vi "GetPicture.vi"(8 "ErrorIn":errorcluster, 11 "OpenCVCamIn":refnum<class "OpenCVCam.lvclass">) -> (0 "ErrorOut":errorcluster, 2 "2D Picture":picture, 3 "OpenCVCamOut":refnum<class "OpenCVCam.lvclass">)   [LabVIEW 2021, in "OpenCVCam.lvclass"]
uses:
  OpenCVCam.lvclass
  C:/Localdata/Projects/TriekselSoft/TriekselsoftApplicationFramework/Source/.Externals/Library_TAF/YActor/YActor.lvclass
  .Externals/Library_TAF/YActor/YActor.lvclass/YActor.ctl
  .Externals/Library_TAF/YActor/ExeCmd_sync.vi
  788cf652-cfa8-44ab-bf5d-4ff5bf462e4f.vi
  .Externals/Library_TAF/YActor/private/SendCommand.vi
  .Externals/Library_TAF/YActor/private/WaitForReply.vi
  .Externals/Library_TAF/YActor/private/CreateLocalVI.vi
  .Externals/Library_TAF/YActor/private/ExeuteInlineVI.vi
  .Externals/Library_TAF/YActor/private/GetRemoteVIRef.vi
  .Externals/Library_TAF/YActor/private/GetNameOfVI.vi
  .Externals/Library_TAF/YActor/QuickCast.vi
  .Externals/Library_TAF/YActor/private/VINameProperty.vi
  .Externals/Library_TAF/YActor/private/MessageCounter.vi
  .Externals/Library_TAF/YActor/InlineReferencePool.vi
  .Externals/Library_TAF/YActor/private/ExecuteVI.vi
  .Externals/Library_TAF/YActor/YActor.lvclass
  C:/Localdata/Projects/TriekselSoft/TriekselsoftApplicationFramework/Source/.Externals/Library_TAF/YAFTAF/YAFTAF.lvclass
  C:/Localdata/Projects/TriekselSoft/TriekselsoftApplicationFramework/Source/.Externals/Interface_UserInterface_IFrontPanel/IFrontPanel/IFrontPanel.lvclass
  C:/Localdata/Projects/TriekselSoft/TriekselsoftApplicationFramework/Source/.Externals/Interface_TAF_IInterface/IInterface/IInterface.lvclass
  C:/Localdata/Projects/TriekselSoft/TriekselsoftApplicationFramework/Source/.Externals/Interface_Object_ICreateDestroy/ICreateDestroy/ICreateDestroy.lvclass
  C:/Localdata/Projects/TriekselSoft/TriekselsoftApplicationFramework/Source/.Externals/Interface_Object_IPersistentData/IPersistentData/IPersistentData.lvclass
  C:/Localdata/Projects/TriekselSoft/TriekselsoftApplicationFramework/Source/.Externals/Interface_TAF_ITAFObject/ITAFObject/ITAFObject.lvclass
  C:/Localdata/Projects/TriekselSoft/TriekselsoftApplicationFramework/Source/YAFTAFObjects/OpenCVCam/OpenCVCam.lvclass
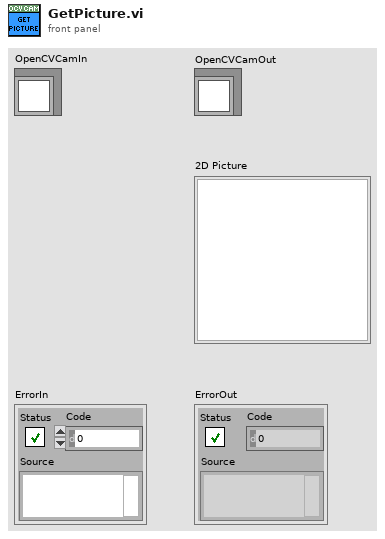
[diagram p1: front panel]
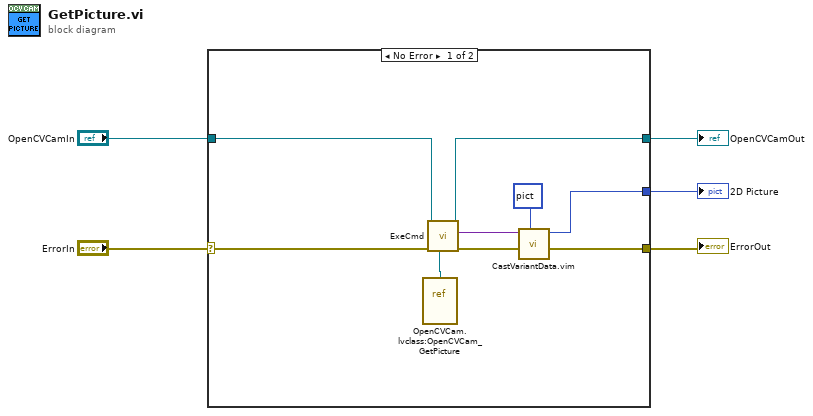
[diagram p0: block diagram]
diagram:
  n1 = case shown="No Error" "ErrorIn" {
    selector: "ErrorIn" -> [w14 w16]
    tunnel: [w12 w16] -> w4
    tunnel: [w7 w15] -> w2
    tunnel: "OpenCVCamIn" -> [w6 w15]
    tunnel: [w10 _] -> w1
    frame No Error {
      n2 = vi-ref "OpenCVCam.lvclass:OpenCVCam_GetPicture.vi"() -> (w11:refnum<vi>)
      n3 = call-poly "ExeCmd.vi"("CmdVIRef"=w11, "ErrorIn"=w14, "YActorIn"=w6) -> ("ErrorOut"=w13:errorcluster, "ReplyData"=w8:variant, "YActorOut"=w7:refnum<class "OpenCVCam.lvclass">)  [unwired: 6 in]
      n4 = call "CastVariantData.vim"("Type"=picture data[5B] ("2D Picture"), "ErrorIn"=w13, "DataIn"=w8) -> ("ErrorOut"=w12:errorcluster, "DataOut"=w10:picture)  [unwired: 7 in]
    }
    frame Error {
    }
  }
  "ErrorOut" <- w4
  "OpenCVCamOut" <- w2
  "2D Picture" <- w1
